vi "Product model selection.vi"(8 "error in (no error)":errorcluster caption="错误输入（无错误）") -> (0 "error in (no error) 2":errorcluster caption="错误输入（无错误）")   [LabVIEW 2017]
uses:
  Picture/SaveButtom.ctl
  Global System.vi
panel:
  out "路径输出":path
  out "添加的路径":path
  in  "Vision Paramter Save Buttom":T1
  out "system time":string
  in  "取消按钮":bool
  in  "确定按钮":bool
  in  "产品处理流程":string(tree)
  in  "产品型号选择":string(combo)
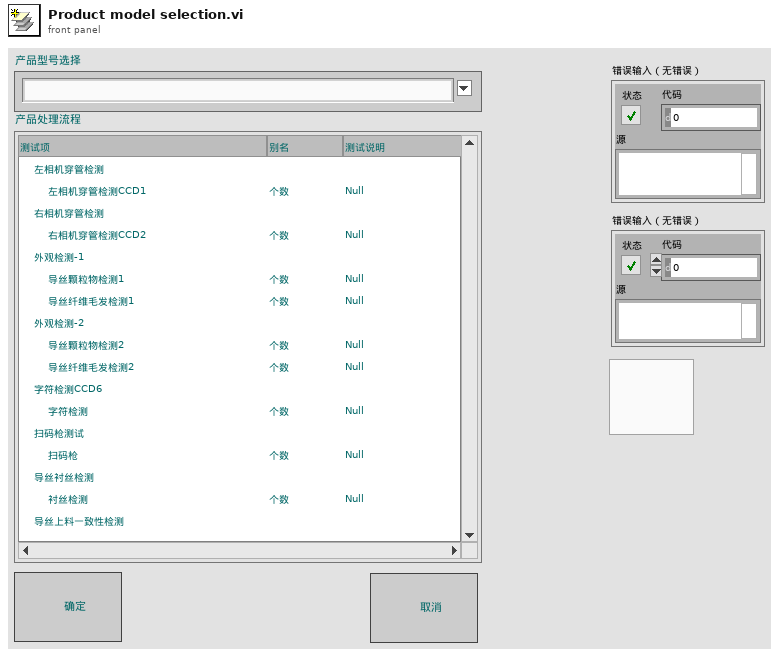
[diagram p1: front panel]
types:
  T1 = typedef "SaveButtom.ctl" = bool
  T2 = cluster{"index":i32, "this vi":refnum<vi>, "error out":errorcluster}
  T3 = cluster{"master data":string, "priority":u16, "secondary data":string[]}
  T4 = cluster{"case name":string[], "queue array":refnum<queue>[]}
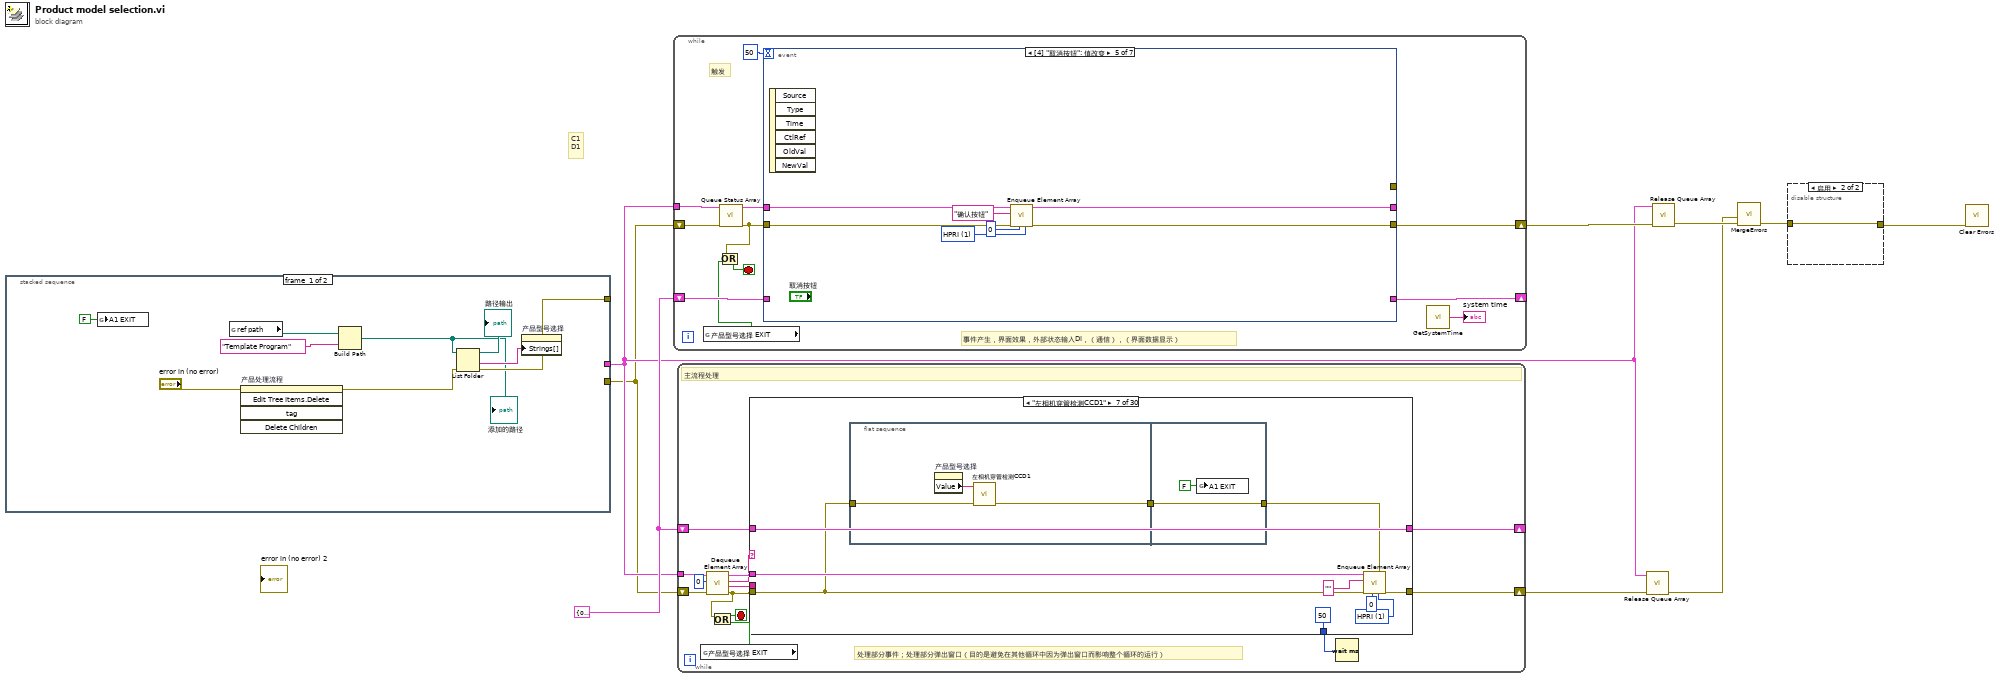
[diagram p0: block diagram]
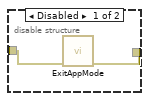
[diagram p2: hidden frame]
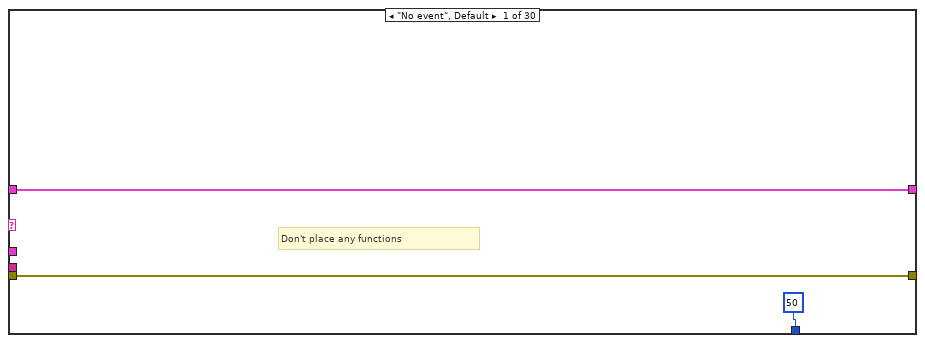
[diagram p3: hidden frame]
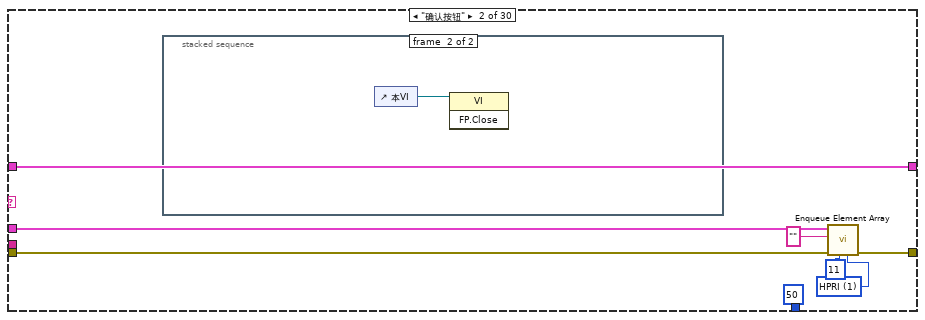
[diagram p4: hidden frame]
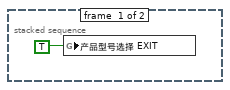
[diagram p5: hidden frame]
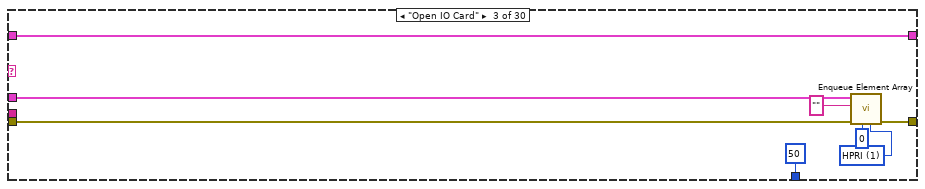
[diagram p6: hidden frame]
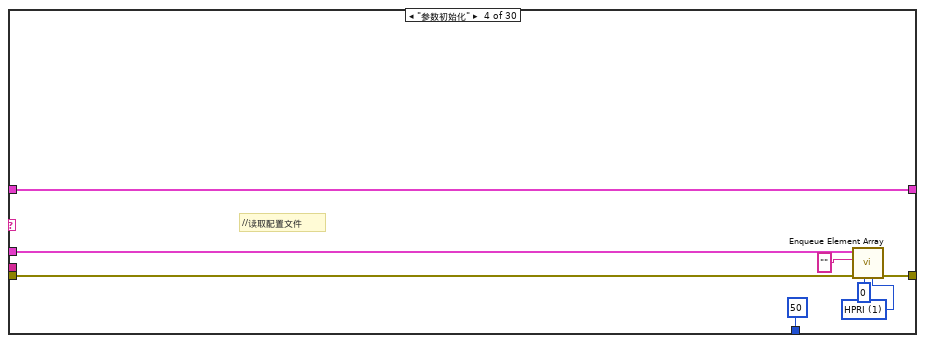
[diagram p7: hidden frame]
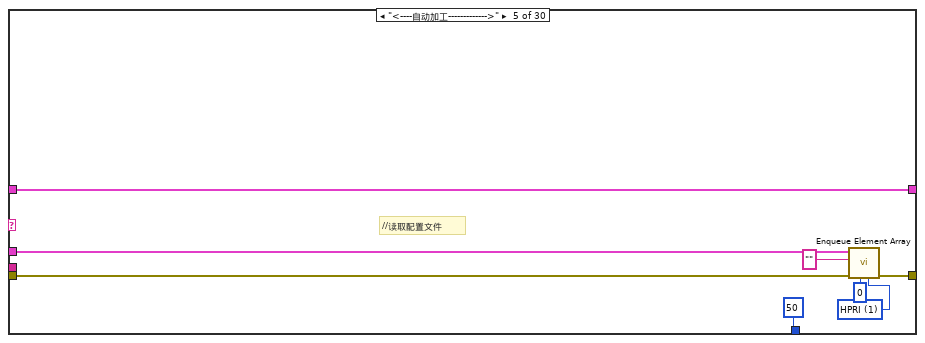
[diagram p8: hidden frame]
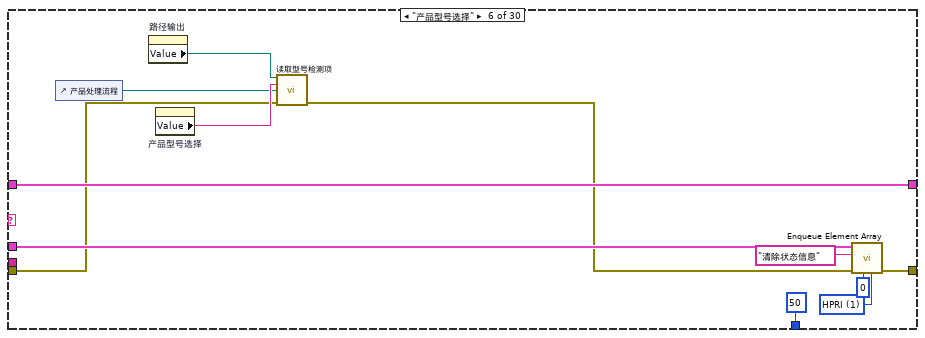
[diagram p9: hidden frame]
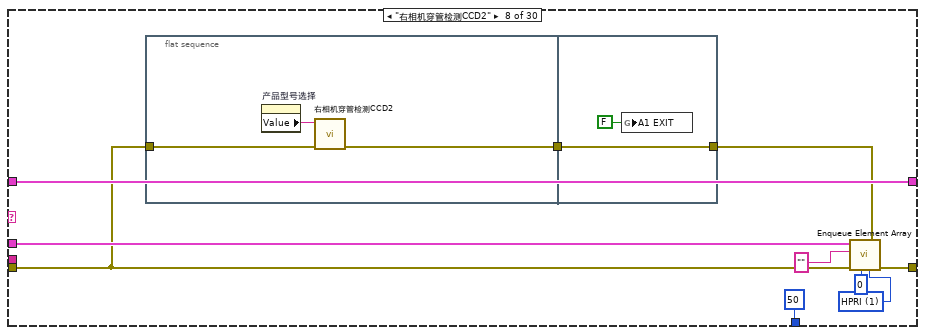
[diagram p10: hidden frame]
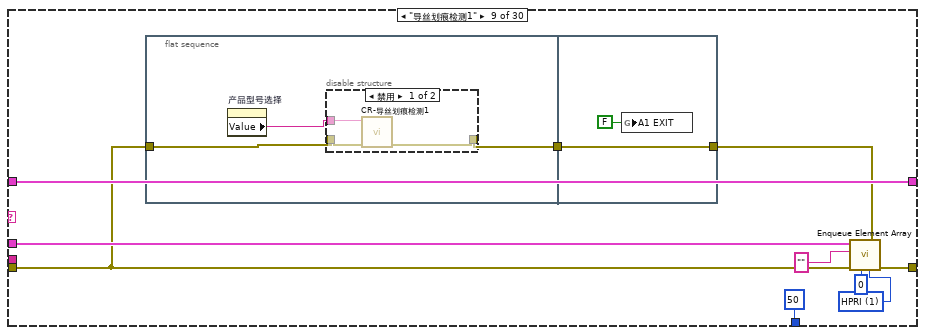
[diagram p11: hidden frame]
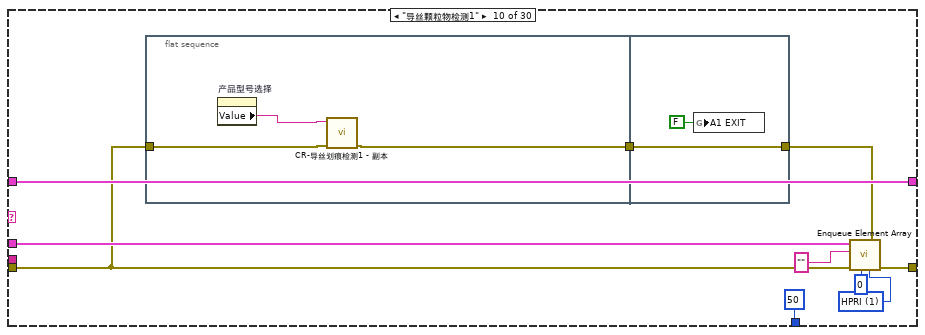
[diagram p13: hidden frame]
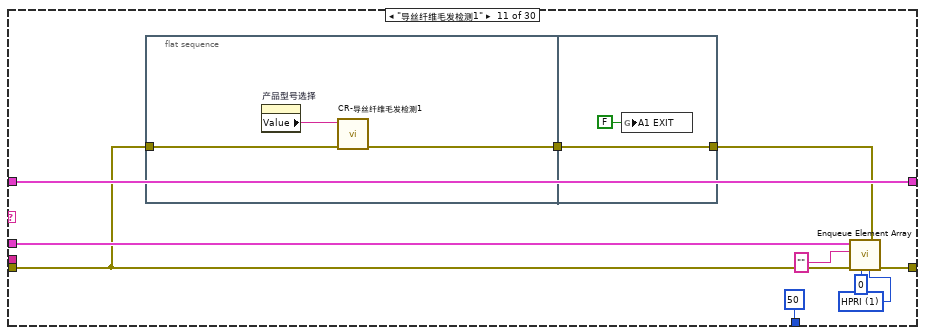
[diagram p14: hidden frame]
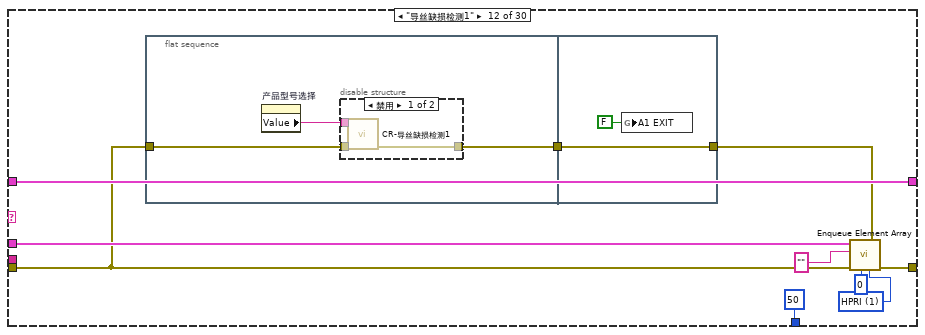
[diagram p15: hidden frame]
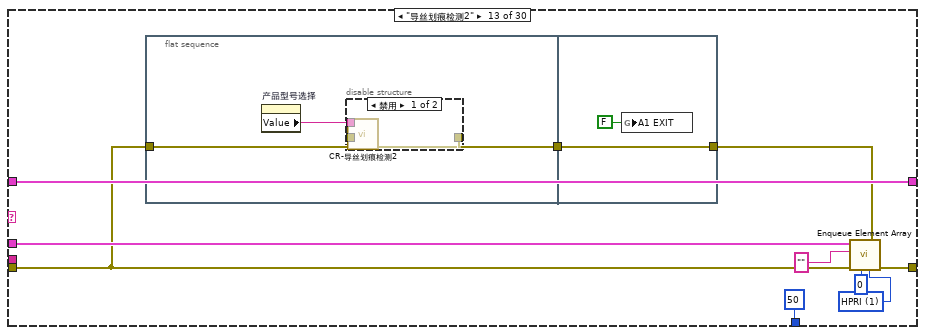
[diagram p17: hidden frame]
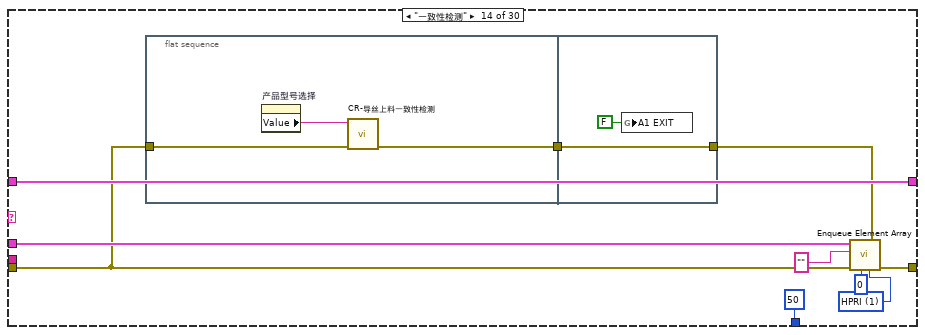
[diagram p19: hidden frame]
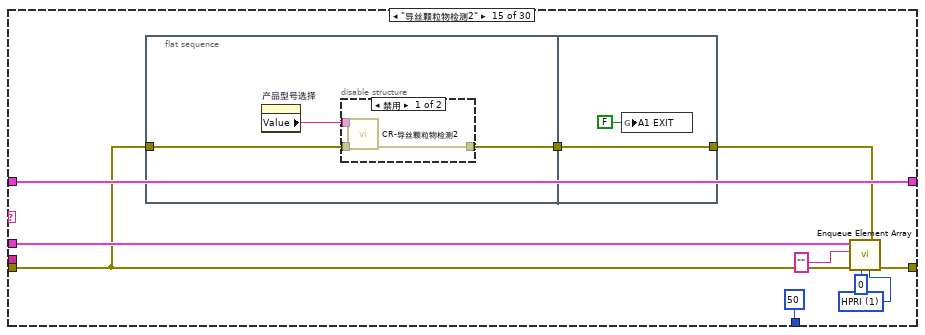
[diagram p20: hidden frame]
diagram:
  w5 = T2 {"index"=0, "this vi"=refnum, "error out"={"status"=FALSE, "code"=0, "source"=""}} ("parameter buffer")
  # "C1\nD1"
  n1 = stacked-sequence {
    tunnel: [w15 _] -> _
    tunnel: [_ w20] -> w1
    tunnel: [_ w19] -> w2
    frame #0 {
      n2 = global write "Global System.vi" "A1 EXIT"(FALSE ("A1 EXIT")) -> ()
      n3 = global read "Global System.vi" "ref path"() -> (w16:path)
      n4 = invoke on="产品处理流程" class="Tree (严格)" method="Edit Tree Items.Delete"(error in="error in (no error)") -> (error out=w11:errorcluster)  [unwired: 4 in, 4 out]
      n5 = Build Path(base path=w16, name or relative path="Template Program" ("名称或相对路径")) -> (appended path=w10:path)
      "添加的路径" <- w10
      n6 = List Folder(path=w10, error in=w11) -> (path out=→"路径输出":path, folder names=w18:string[], error out=w15:errorcluster)  [unwired: 2 in, 1 out]
      n7 = property on="产品型号选择" class="CmbBox"("Strings[]"=w18) -> ()  [unwired: 2 in, 2 out]
    }
    frame #1 {
      w28 = string[] ["comm queue1", "data queue 11", "data queue 12", "data queue 13", "data queue 14"]  # queue name
      w29 = 4  # queue num
      w30 = T3 {"master data"="", "priority"=0, "secondary data"=[]}  # element data type
      n8 = call "Obtain Queue Array.vi"("queue name"=w28, "element data type"=w30, "queue num"=w29) -> ("error out"=w24:errorcluster, "queue out"=w25:T4)  [unwired: 2 in, 1 out]
      n9 = call "Enqueue Element Array.vi"("queue index"=0, "error in"=w24, "master data"="参数初始化", "queue in"=w25) -> ("error out"=w23:errorcluster, "queue out"=w22:T4)  [unwired: 6 in]
      n10 = disable-structure shown="启用" {
        disable-tunnel: w23 -> [w36 w37]
        disable-tunnel: w22 -> [w35 w38]
        disable-tunnel: "Loading Variable" ("master data") -> [w34 _]
        disable-tunnel: [w32 w37] -> w20
        disable-tunnel: [w31 w38] -> w19
        frame Disabled {
          n11 = call "Enqueue Element Array.vi"("queue index"=12, "error in"=w36, "master data"=w34, "queue in"=w35) -> ("error out"=w32:errorcluster, "queue out"=w31:T4)  [unwired: 6 in]
        }
        frame Enabled {
        }
      }
    }
  }
  n12 = while {
    shift-right: [w42] -> w6
    shift-left: w1 -> [w46]
    shift-right: [w44] -> _
    shift-left: w5 -> [w45]
    tunnel: w2 -> [w48]
    stop <- w39 stop-if-true
    # "触发"
    # "事件产生，界面效果，外部状态输入DI，（通信），（界面数据显示）"
    n13 = global read "Global System.vi" "产品型号选择 EXIT"() -> (w40:bool)
    n14 = call "Queue Status Array.vi"("error in (no error)"=w46, "queue in"=w48) -> ("error out"=w41:errorcluster, "queue out"=w43:T4)  [unwired: 4 in]
    n15 = Or(x=w41, y=w40) -> (x .or. y?=w39:bool)
    n16 = event shown="[4] \"取消按钮\": 值改变" {
      selector: _ -> [_ _ _ _ _ _ _]
      dyn-events: _ -> [_ _ _ _ _ _ _]
      timeout: 50 -> [_ _ _ _ _ _ _]
      tunnel: w45 -> [w53 w61 _ _ _ _ _]
      tunnel: [w53 w61 _ _ _ _ _] -> w44
      tunnel: [errorcluster {"status"=FALSE, "code"=0, "source"=""} ("error out") _ _ _ _ _ _] -> _
      tunnel: w43 -> [w51 w60 w66 w73 w80 w87 w95]
      tunnel: w41 -> [w50 w59 w65 w72 w79 w86 w94]
      tunnel: [w50 w58 w63 w70 w77 w84 w92] -> w42
      tunnel: [w51 w57 w64 w71 w78 w85 w93] -> _
      event Timeout {
        # "不要在事件结构里面放入\"弹出窗口\"这样的VI保证该循环畅通无阻。"
        n17 = event-data() -> ()  [unwired: 1 in, 1 out]
      }
      event Panel Close? {
        w55 = u16 1 items=["HPRI"=1, "LPRI"=0] ("priority")
        n18 = event-data() -> ()  [unwired: 1 in, 4 out]
        n19 = call "Enqueue Element Array.vi"("priority"=w55, "queue index"=0, "error in"=w59, "master data"="*Exit application", "queue in"=w60) -> ("error out"=w58:errorcluster, "queue out"=w57:T4)  [unwired: 5 in]
        n20 = event-data("Discard?"=TRUE) -> ()  [unwired: 1 in, 1 out]
      }
      event Value Change {
        w68 = u16 1 items=["HPRI"=1, "LPRI"=0] ("priority")
        n21 = event-data() -> ()  [unwired: 1 in, 6 out]
        n22 = call "Enqueue Element Array.vi"("priority"=w68, "queue index"=0, "error in"=w65, "master data"="Vision Paramter Save", "queue in"=w66) -> ("error out"=w63:errorcluster, "queue out"=w64:T4)  [unwired: 5 in]
      }
      event "确定按钮": Value Change {
        w75 = u16 1 items=["HPRI"=1, "LPRI"=0] ("priority")
        n23 = event-data() -> ()  [unwired: 1 in, 6 out]
        n24 = call "Enqueue Element Array.vi"("priority"=w75, "queue index"=0, "error in"=w72, "master data"="确认按钮", "queue in"=w73) -> ("error out"=w70:errorcluster, "queue out"=w71:T4)  [unwired: 5 in]
      }
      event "取消按钮": Value Change {
        w82 = u16 1 items=["HPRI"=1, "LPRI"=0] ("priority")
        n25 = event-data() -> ()  [unwired: 1 in, 6 out]
        n26 = call "Enqueue Element Array.vi"("priority"=w82, "queue index"=0, "error in"=w79, "master data"="确认按钮", "queue in"=w80) -> ("error out"=w77:errorcluster, "queue out"=w78:T4)  [unwired: 5 in]
      }
      event "产品型号选择": Value Change {
        w89 = u16 1 items=["HPRI"=1, "LPRI"=0] ("priority")
        n27 = event-data() -> ()  [unwired: 1 in, 6 out]
        n28 = call "Enqueue Element Array.vi"("priority"=w89, "queue index"=0, "error in"=w86, "master data"="产品型号选择", "queue in"=w87) -> ("error out"=w84:errorcluster, "queue out"=w85:T4)  [unwired: 5 in]
      }
      event "产品处理流程": Value Change {
        n29 = event-data() -> ("NewVal"=w91:string)  [unwired: 1 in, 5 out]
        n30 = case shown="\"一致性检测\"" w91 {
          tunnel: w95 -> [w97 w104 w111 w118 w125 w132 w139 w146 w153 w160 w167 w174 w181 w188 w195 w202 w209 w216 w223]
          tunnel: w94 -> [w96 w103 w110 w117 w124 w131 w138 w145 w152 w159 w166 w173 w180 w187 w194 w201 w208 w215 w222]
          tunnel: [w97 w102 w109 w116 w123 w130 w137 w144 w151 w158 w165 w172 w179 w186 w193 w200 w207 w214 w221] -> w93
          tunnel: [w96 w101 w108 w115 w122 w129 w136 w143 w150 w157 w164 w171 w178 w185 w192 w199 w206 w213 w220] -> w92
          frame "假", Default {
          }
          frame "左相机穿管检测CCD1" {
            w99 = u16 1 items=["HPRI"=1, "LPRI"=0] ("priority")
            n31 = call "Enqueue Element Array.vi"("priority"=w99, "queue index"=0, "error in"=w103, "master data"="左相机穿管检测CCD1", "queue in"=w104) -> ("error out"=w101:errorcluster, "queue out"=w102:T4)  [unwired: 5 in]
          }
          frame "右相机穿管检测CCD2" {
            w106 = u16 1 items=["HPRI"=1, "LPRI"=0] ("priority")
            n32 = call "Enqueue Element Array.vi"("priority"=w106, "queue index"=0, "error in"=w110, "master data"="右相机穿管检测CCD2", "queue in"=w111) -> ("error out"=w108:errorcluster, "queue out"=w109:T4)  [unwired: 5 in]
          }
          frame "导丝划痕检测1" {
            w113 = u16 1 items=["HPRI"=1, "LPRI"=0] ("priority")
            n33 = call "Enqueue Element Array.vi"("priority"=w113, "queue index"=0, "error in"=w117, "master data"="导丝划痕检测1", "queue in"=w118) -> ("error out"=w115:errorcluster, "queue out"=w116:T4)  [unwired: 5 in]
          }
          frame "导丝颗粒物检测1" {
            w120 = u16 1 items=["HPRI"=1, "LPRI"=0] ("priority")
            n34 = call "Enqueue Element Array.vi"("priority"=w120, "queue index"=0, "error in"=w124, "master data"="导丝颗粒物检测1", "queue in"=w125) -> ("error out"=w122:errorcluster, "queue out"=w123:T4)  [unwired: 5 in]
          }
          frame "导丝纤维毛发检测1" {
            w127 = u16 1 items=["HPRI"=1, "LPRI"=0] ("priority")
            n35 = call "Enqueue Element Array.vi"("priority"=w127, "queue index"=0, "error in"=w131, "master data"="导丝纤维毛发检测1", "queue in"=w132) -> ("error out"=w129:errorcluster, "queue out"=w130:T4)  [unwired: 5 in]
          }
          frame "导丝缺损检测1" {
            w134 = u16 1 items=["HPRI"=1, "LPRI"=0] ("priority")
            n36 = call "Enqueue Element Array.vi"("priority"=w134, "queue index"=0, "error in"=w138, "master data"="导丝缺损检测1", "queue in"=w139) -> ("error out"=w136:errorcluster, "queue out"=w137:T4)  [unwired: 5 in]
          }
          frame "导丝划痕检测2" {
            w141 = u16 1 items=["HPRI"=1, "LPRI"=0] ("priority")
            n37 = call "Enqueue Element Array.vi"("priority"=w141, "queue index"=0, "error in"=w145, "master data"="导丝划痕检测2", "queue in"=w146) -> ("error out"=w143:errorcluster, "queue out"=w144:T4)  [unwired: 5 in]
          }
          frame "导丝颗粒物检测2" {
            w148 = u16 1 items=["HPRI"=1, "LPRI"=0] ("priority")
            n38 = call "Enqueue Element Array.vi"("priority"=w148, "queue index"=0, "error in"=w152, "master data"="导丝颗粒物检测2", "queue in"=w153) -> ("error out"=w150:errorcluster, "queue out"=w151:T4)  [unwired: 5 in]
          }
          frame "导丝纤维毛发检测2" {
            w155 = u16 1 items=["HPRI"=1, "LPRI"=0] ("priority")
            n39 = call "Enqueue Element Array.vi"("priority"=w155, "queue index"=0, "error in"=w159, "master data"="导丝纤维毛发检测2", "queue in"=w160) -> ("error out"=w157:errorcluster, "queue out"=w158:T4)  [unwired: 5 in]
          }
          frame "导丝缺损检测2" {
            w162 = u16 1 items=["HPRI"=1, "LPRI"=0] ("priority")
            n40 = call "Enqueue Element Array.vi"("priority"=w162, "queue index"=0, "error in"=w166, "master data"="导丝缺损检测2", "queue in"=w167) -> ("error out"=w164:errorcluster, "queue out"=w165:T4)  [unwired: 5 in]
          }
          frame "导丝划痕检测3" {
            w169 = u16 1 items=["HPRI"=1, "LPRI"=0] ("priority")
            n41 = call "Enqueue Element Array.vi"("priority"=w169, "queue index"=0, "error in"=w173, "master data"="导丝划痕检测3", "queue in"=w174) -> ("error out"=w171:errorcluster, "queue out"=w172:T4)  [unwired: 5 in]
          }
          frame "导丝颗粒物检测3" {
            w176 = u16 1 items=["HPRI"=1, "LPRI"=0] ("priority")
            n42 = call "Enqueue Element Array.vi"("priority"=w176, "queue index"=0, "error in"=w180, "master data"="导丝颗粒物检测3", "queue in"=w181) -> ("error out"=w178:errorcluster, "queue out"=w179:T4)  [unwired: 5 in]
          }
          frame "导丝纤维毛发检测3" {
            w183 = u16 1 items=["HPRI"=1, "LPRI"=0] ("priority")
            n43 = call "Enqueue Element Array.vi"("priority"=w183, "queue index"=0, "error in"=w187, "master data"="导丝纤维毛发检测3", "queue in"=w188) -> ("error out"=w185:errorcluster, "queue out"=w186:T4)  [unwired: 5 in]
          }
          frame "导丝缺损检测3" {
            w190 = u16 1 items=["HPRI"=1, "LPRI"=0] ("priority")
            n44 = call "Enqueue Element Array.vi"("priority"=w190, "queue index"=0, "error in"=w194, "master data"="导丝缺损检测3", "queue in"=w195) -> ("error out"=w192:errorcluster, "queue out"=w193:T4)  [unwired: 5 in]
          }
          frame "字符检测" {
            w197 = u16 1 items=["HPRI"=1, "LPRI"=0] ("priority")
            n45 = call "Enqueue Element Array.vi"("priority"=w197, "queue index"=0, "error in"=w201, "master data"="字符检测", "queue in"=w202) -> ("error out"=w199:errorcluster, "queue out"=w200:T4)  [unwired: 5 in]
          }
          frame "扫码枪" {
            w204 = u16 1 items=["HPRI"=1, "LPRI"=0] ("priority")
            n46 = call "Enqueue Element Array.vi"("priority"=w204, "queue index"=0, "error in"=w208, "master data"="扫码枪扫码", "queue in"=w209) -> ("error out"=w206:errorcluster, "queue out"=w207:T4)  [unwired: 5 in]
          }
          frame "衬丝检测" {
            w211 = u16 1 items=["HPRI"=1, "LPRI"=0] ("priority")
            n47 = call "Enqueue Element Array.vi"("priority"=w211, "queue index"=0, "error in"=w215, "master data"="衬丝检测", "queue in"=w216) -> ("error out"=w213:errorcluster, "queue out"=w214:T4)  [unwired: 5 in]
          }
          frame "一致性检测" {
            w218 = u16 1 items=["HPRI"=1, "LPRI"=0] ("priority")
            n48 = call "Enqueue Element Array.vi"("priority"=w218, "queue index"=0, "error in"=w222, "master data"="一致性检测", "queue in"=w223) -> ("error out"=w220:errorcluster, "queue out"=w221:T4)  [unwired: 5 in]
          }
        }
      }
    }
    n49 = call "GetSystemTime.vi"() -> ("date/time string"=→"system time":string)  [unwired: 7 in]
  }
  n50 = while {
    shift-right: [w236] -> w4
    shift-left: w1 -> [w227]
    shift-right: [w233] -> _
    shift-left: w5 -> [w234]
    tunnel: w2 -> [w229]
    stop <- w224 stop-if-true
    # "处理部分事件；处理部分弹出窗口（目的是避免在其他循环中因为弹出窗口而影响整个循环的运行）"
    # "主流程处理"
    n51 = global read "Global System.vi" "产品型号选择 EXIT"() -> (w225:bool)
    n52 = call "Dequeue Element Array.vi"("queue in"=w229, "queue index"=0, "error in"=w227) -> ("queue out"=w232:T4, "master data"=w231:string, "secondary data"=w230:string[], "error out"=w226:errorcluster)  [unwired: 2 in, 1 out]
    n53 = Or(x=w226, y=w225) -> (x .or. y?=w224:bool)
    n54 = case shown="\"左相机穿管检测CCD1\"" w231 {
      tunnel: w232 -> [_ w246 w256 w264 w272 w279 w294 w309 w324 w342 w357 w372 w390 w408 w423 w441 w459 w477 w495 w513 w531 w549 w564 w579 w592 w600 w608 w616 w624 w630]
      tunnel: w226 -> [w238 w242 w252 w261 w268 w275 w288 w303 w318 w336 w351 w366 w384 w402 w417 w435 w453 w471 w489 w507 w525 w543 w558 w573 w587 w596 w604 w612 w620 w627]
      tunnel: [w238 w245 w255 w263 w271 w284 w293 w308 w323 w341 w356 w371 w389 w407 w422 w440 w458 w476 w494 w512 w530 w548 w563 w578 w591 w599 w607 w615 w623 w638] -> w236
      tunnel: [50 50 50 50 50 50 50 50 50 50 50 50 50 50 50 50 50 50 50 50 50 50 50 50 50 50 50 50 50 50] -> w235
      tunnel: w234 -> [w239 w243 w253 w258 w269 w280 w289 w304 w319 w337 w352 w367 w385 w403 w418 w436 w454 w472 w490 w508 w526 w544 w559 w574 w586 w597 w605 w613 w621 w636]
      tunnel: [w239 w243 w253 w258 w269 w280 w289 w304 w319 w337 w352 w367 w385 w403 w418 w436 w454 w472 w490 w508 w526 w544 w559 w574 w586 w597 w605 w613 w621 w636] -> w233
      tunnel: w230 -> [_ _ _ _ _ _ _ _ _ _ _ _ _ _ _ _ _ _ _ _ _ _ _ _ _ _ _ _ _ _]
      frame "No event", Default {
        # "Don't place any functions"
      }
      frame "确认按钮" {
        w240 = u16 1 items=["HPRI"=1, "LPRI"=0] ("priority")
        n55 = stacked-sequence {
          frame #0 {
            n56 = global write "Global System.vi" "产品型号选择 EXIT"(TRUE ("EXIT")) -> ()
          }
          frame #1 {
            n57 = control-ref of="本VI"() -> (w249:refnum<vi>)
            n58 = invoke class="VI" method="FP.Close"(reference=w249) -> ()  [unwired: 2 in, 3 out]
          }
        }
        n59 = call "Enqueue Element Array.vi"("priority"=w240, "queue index"=11, "error in"=w242, "master data"="" ("Element 1"), "queue in"=w246) -> ("error out"=w245:errorcluster)  [unwired: 5 in, 1 out]
      }
      frame "Open IO Card" {
        w250 = u16 1 items=["HPRI"=1, "LPRI"=0] ("priority")
        n60 = call "Enqueue Element Array.vi"("priority"=w250, "queue index"=0, "error in"=w252, "master data"="" ("Element 1"), "queue in"=w256) -> ("error out"=w255:errorcluster)  [unwired: 5 in, 1 out]
      }
      frame "参数初始化" {
        w259 = u16 1 items=["HPRI"=1, "LPRI"=0] ("priority")
        # "//读取配置文件"
        n61 = call "Enqueue Element Array.vi"("priority"=w259, "queue index"=0, "error in"=w261, "master data"="" ("Element 1"), "queue in"=w264) -> ("error out"=w263:errorcluster)  [unwired: 5 in, 1 out]
      }
      frame "<----自动加工------------->" {
        w266 = u16 1 items=["HPRI"=1, "LPRI"=0] ("priority")
        # "//读取配置文件"
        n62 = call "Enqueue Element Array.vi"("priority"=w266, "queue index"=0, "error in"=w268, "master data"="" ("Element 1"), "queue in"=w272) -> ("error out"=w271:errorcluster)  [unwired: 5 in, 1 out]
      }
      frame "产品型号选择" {
        w281 = u16 1 items=["HPRI"=1, "LPRI"=0] ("priority")
        n63 = control-ref of="产品处理流程"() -> (w276:refnum<vi>)
        n64 = property on="路径输出" class="Path"() -> ("Value"=w278:path)  [unwired: 2 in, 2 out]
        n65 = property on="产品型号选择" class="CmbBox"() -> ("Value"=w277:string)  [unwired: 2 in, 2 out]
        n66 = call "读取型号检测项.vi"("产品型号路径"=w278, "产品型号"=w277, "树形List"=w276, "error in (no error)"=w275) -> ("error out"=w274:errorcluster)  [unwired: 11 in]
        n67 = call "Enqueue Element Array.vi"("priority"=w281, "queue index"=0, "error in"=w274, "master data"="清除状态信息" ("Element 1"), "queue in"=w279) -> ("error out"=w284:errorcluster)  [unwired: 5 in, 1 out]
      }
      frame "左相机穿管检测CCD1" {
        w290 = u16 1 items=["HPRI"=1, "LPRI"=0] ("priority")
        n68 = flat-sequence {
          tunnel: w288 -> [w298]
          tunnel: [w297] -> w286
          tunnel: [w299] -> w287
          tunnel: w286 -> [w299]
          frame #0 {
            n69 = property on="产品型号选择" class="CmbBox"() -> ("Value"=w296:string)  [unwired: 2 in, 2 out]
            n70 = call "左相机穿管检测CCD1.vi"("error in (no error)"=w298, "名称或相对路径"=w296) -> ("error in (no error) 2"=w297:errorcluster)  [unwired: 9 in]
          }
          frame #1 {
            n71 = global write "Global System.vi" "A1 EXIT"(FALSE ("A1 EXIT")) -> ()
          }
        }
        n72 = call "Enqueue Element Array.vi"("priority"=w290, "device error in"=w287, "queue index"=0, "error in"=w288, "master data"="" ("Element 1"), "queue in"=w294) -> ("error out"=w293:errorcluster)  [unwired: 4 in, 1 out]
      }
      frame "右相机穿管检测CCD2" {
        w305 = u16 1 items=["HPRI"=1, "LPRI"=0] ("priority")
        n73 = flat-sequence {
          tunnel: w303 -> [w313]
          tunnel: [w312] -> w301
          tunnel: [w314] -> w302
          tunnel: w301 -> [w314]
          frame #0 {
            n74 = property on="产品型号选择" class="CmbBox"() -> ("Value"=w311:string)  [unwired: 2 in, 2 out]
            n75 = call "右相机穿管检测CCD2.vi"("error in (no error)"=w313, "名称或相对路径"=w311) -> ("error in (no error) 2"=w312:errorcluster)  [unwired: 9 in]
          }
          frame #1 {
            n76 = global write "Global System.vi" "A1 EXIT"(FALSE ("A1 EXIT")) -> ()
          }
        }
        n77 = call "Enqueue Element Array.vi"("priority"=w305, "device error in"=w302, "queue index"=0, "error in"=w303, "master data"="" ("Element 1"), "queue in"=w309) -> ("error out"=w308:errorcluster)  [unwired: 4 in, 1 out]
      }
      frame "导丝划痕检测1" {
        w320 = u16 1 items=["HPRI"=1, "LPRI"=0] ("priority")
        n78 = flat-sequence {
          tunnel: w318 -> [w328]
          tunnel: [w327] -> w316
          tunnel: [w332] -> w317
          tunnel: w316 -> [w332]
          frame #0 {
            n79 = property on="产品型号选择" class="CmbBox"() -> ("Value"=w326:string)  [unwired: 2 in, 2 out]
            n80 = disable-structure shown="禁用" {
              disable-tunnel: w328 -> [w331 _]
              disable-tunnel: [w330 _] -> w327
              disable-tunnel: w326 -> [w329 _]
              frame Disabled {
                n81 = call "CR-导丝划痕检测1.vi"("error in (no error)"=w331, "名称或相对路径"=w329) -> ("error in (no error) 2"=w330:errorcluster)  [unwired: 9 in]
              }
              frame Enabled {
              }
            }
          }
          frame #1 {
            n82 = global write "Global System.vi" "A1 EXIT"(FALSE ("A1 EXIT")) -> ()
          }
        }
        n83 = call "Enqueue Element Array.vi"("priority"=w320, "device error in"=w317, "queue index"=0, "error in"=w318, "master data"="" ("Element 1"), "queue in"=w324) -> ("error out"=w323:errorcluster)  [unwired: 4 in, 1 out]
      }
      frame "导丝颗粒物检测1" {
        w338 = u16 1 items=["HPRI"=1, "LPRI"=0] ("priority")
        n84 = flat-sequence {
          tunnel: w336 -> [w346]
          tunnel: [w345] -> w334
          tunnel: [w347] -> w335
          tunnel: w334 -> [w347]
          frame #0 {
            n85 = property on="产品型号选择" class="CmbBox"() -> ("Value"=w344:string)  [unwired: 2 in, 2 out]
            n86 = call "CR-导丝划痕检测1 - 副本.vi"("error in (no error)"=w346, "名称或相对路径"=w344) -> ("error in (no error) 2"=w345:errorcluster)  [unwired: 9 in]
          }
          frame #1 {
            n87 = global write "Global System.vi" "A1 EXIT"(FALSE ("A1 EXIT")) -> ()
          }
        }
        n88 = call "Enqueue Element Array.vi"("priority"=w338, "device error in"=w335, "queue index"=0, "error in"=w336, "master data"="" ("Element 1"), "queue in"=w342) -> ("error out"=w341:errorcluster)  [unwired: 4 in, 1 out]
      }
      frame "导丝纤维毛发检测1" {
        w353 = u16 1 items=["HPRI"=1, "LPRI"=0] ("priority")
        n89 = flat-sequence {
          tunnel: w351 -> [w361]
          tunnel: [w360] -> w349
          tunnel: [w362] -> w350
          tunnel: w349 -> [w362]
          frame #0 {
            n90 = property on="产品型号选择" class="CmbBox"() -> ("Value"=w359:string)  [unwired: 2 in, 2 out]
            n91 = call "CR-导丝纤维毛发检测1.vi"("error in (no error)"=w361, "名称或相对路径"=w359) -> ("error in (no error) 2"=w360:errorcluster)  [unwired: 9 in]
          }
          frame #1 {
            n92 = global write "Global System.vi" "A1 EXIT"(FALSE ("A1 EXIT")) -> ()
          }
        }
        n93 = call "Enqueue Element Array.vi"("priority"=w353, "device error in"=w350, "queue index"=0, "error in"=w351, "master data"="" ("Element 1"), "queue in"=w357) -> ("error out"=w356:errorcluster)  [unwired: 4 in, 1 out]
      }
      frame "导丝缺损检测1" {
        w368 = u16 1 items=["HPRI"=1, "LPRI"=0] ("priority")
        n94 = flat-sequence {
          tunnel: w366 -> [w376]
          tunnel: [w375] -> w364
          tunnel: [w380] -> w365
          tunnel: w364 -> [w380]
          frame #0 {
            n95 = property on="产品型号选择" class="CmbBox"() -> ("Value"=w374:string)  [unwired: 2 in, 2 out]
            n96 = disable-structure shown="禁用" {
              disable-tunnel: w376 -> [w379 _]
              disable-tunnel: [w378 _] -> w375
              disable-tunnel: w374 -> [w377 _]
              frame Disabled {
                n97 = call "CR-导丝缺损检测1.vi"("error in (no error)"=w379, "名称或相对路径"=w377) -> ("error in (no error) 2"=w378:errorcluster)  [unwired: 9 in]
              }
              frame Enabled {
              }
            }
          }
          frame #1 {
            n98 = global write "Global System.vi" "A1 EXIT"(FALSE ("A1 EXIT")) -> ()
          }
        }
        n99 = call "Enqueue Element Array.vi"("priority"=w368, "device error in"=w365, "queue index"=0, "error in"=w366, "master data"="" ("Element 1"), "queue in"=w372) -> ("error out"=w371:errorcluster)  [unwired: 4 in, 1 out]
      }
      frame "导丝划痕检测2" {
        w386 = u16 1 items=["HPRI"=1, "LPRI"=0] ("priority")
        n100 = flat-sequence {
          tunnel: w384 -> [w394]
          tunnel: [w393] -> w382
          tunnel: [w398] -> w383
          tunnel: w382 -> [w398]
          frame #0 {
            n101 = property on="产品型号选择" class="CmbBox"() -> ("Value"=w392:string)  [unwired: 2 in, 2 out]
            n102 = disable-structure shown="禁用" {
              disable-tunnel: w394 -> [w397 _]
              disable-tunnel: [w396 _] -> w393
              disable-tunnel: w392 -> [w395 _]
              frame Disabled {
                n103 = call "CR-导丝划痕检测2.vi"("error in (no error)"=w397, "名称或相对路径"=w395) -> ("error in (no error) 2"=w396:errorcluster)  [unwired: 9 in]
              }
              frame Enabled {
              }
            }
          }
          frame #1 {
            n104 = global write "Global System.vi" "A1 EXIT"(FALSE ("A1 EXIT")) -> ()
          }
        }
        n105 = call "Enqueue Element Array.vi"("priority"=w386, "device error in"=w383, "queue index"=0, "error in"=w384, "master data"="" ("Element 1"), "queue in"=w390) -> ("error out"=w389:errorcluster)  [unwired: 4 in, 1 out]
      }
      frame "一致性检测" {
        w404 = u16 1 items=["HPRI"=1, "LPRI"=0] ("priority")
        n106 = flat-sequence {
          tunnel: w402 -> [w412]
          tunnel: [w411] -> w400
          tunnel: [w413] -> w401
          tunnel: w400 -> [w413]
          frame #0 {
            n107 = property on="产品型号选择" class="CmbBox"() -> ("Value"=w410:string)  [unwired: 2 in, 2 out]
            n108 = call "CR-导丝上料一致性检测.vi"("error in (no error)"=w412, "名称或相对路径"=w410) -> ("error in (no error) 2"=w411:errorcluster)  [unwired: 9 in]
          }
          frame #1 {
            n109 = global write "Global System.vi" "A1 EXIT"(FALSE ("A1 EXIT")) -> ()
          }
        }
        n110 = call "Enqueue Element Array.vi"("priority"=w404, "device error in"=w401, "queue index"=0, "error in"=w402, "master data"="" ("Element 1"), "queue in"=w408) -> ("error out"=w407:errorcluster)  [unwired: 4 in, 1 out]
      }
      frame "导丝颗粒物检测2" {
        w419 = u16 1 items=["HPRI"=1, "LPRI"=0] ("priority")
        n111 = flat-sequence {
          tunnel: w417 -> [w427]
          tunnel: [w426] -> w415
          tunnel: [w431] -> w416
          tunnel: w415 -> [w431]
          frame #0 {
            n112 = property on="产品型号选择" class="CmbBox"() -> ("Value"=w425:string)  [unwired: 2 in, 2 out]
            n113 = disable-structure shown="禁用" {
              disable-tunnel: w427 -> [w430 _]
              disable-tunnel: [w429 _] -> w426
              disable-tunnel: w425 -> [w428 _]
              frame Disabled {
                n114 = call "CR-导丝颗粒物检测2.vi"("error in (no error)"=w430, "名称或相对路径"=w428) -> ("error in (no error) 2"=w429:errorcluster)  [unwired: 9 in]
              }
              frame Enabled {
              }
            }
          }
          frame #1 {
            n115 = global write "Global System.vi" "A1 EXIT"(FALSE ("A1 EXIT")) -> ()
          }
        }
        n116 = call "Enqueue Element Array.vi"("priority"=w419, "device error in"=w416, "queue index"=0, "error in"=w417, "master data"="" ("Element 1"), "queue in"=w423) -> ("error out"=w422:errorcluster)  [unwired: 4 in, 1 out]
      }
      frame "导丝纤维毛发检测2" {
        w437 = u16 1 items=["HPRI"=1, "LPRI"=0] ("priority")
        n117 = flat-sequence {
          tunnel: w435 -> [w445]
          tunnel: [w444] -> w433
          tunnel: [w449] -> w434
          tunnel: w433 -> [w449]
          frame #0 {
            n118 = property on="产品型号选择" class="CmbBox"() -> ("Value"=w443:string)  [unwired: 2 in, 2 out]
            n119 = disable-structure shown="禁用" {
              disable-tunnel: w445 -> [w448 _]
              disable-tunnel: [w447 _] -> w444
              disable-tunnel: w443 -> [w446 _]
              frame Disabled {
                n120 = call "CR-导丝纤维毛发检测2.vi"("error in (no error)"=w448, "名称或相对路径"=w446) -> ("error in (no error) 2"=w447:errorcluster)  [unwired: 9 in]
              }
              frame Enabled {
              }
            }
          }
          frame #1 {
            n121 = global write "Global System.vi" "A1 EXIT"(FALSE ("A1 EXIT")) -> ()
          }
        }
        n122 = call "Enqueue Element Array.vi"("priority"=w437, "device error in"=w434, "queue index"=0, "error in"=w435, "master data"="" ("Element 1"), "queue in"=w441) -> ("error out"=w440:errorcluster)  [unwired: 4 in, 1 out]
      }
      frame "导丝缺损检测2" {
        w455 = u16 1 items=["HPRI"=1, "LPRI"=0] ("priority")
        n123 = flat-sequence {
          tunnel: w453 -> [w463]
          tunnel: [w462] -> w451
          tunnel: [w467] -> w452
          tunnel: w451 -> [w467]
          frame #0 {
            n124 = property on="产品型号选择" class="CmbBox"() -> ("Value"=w461:string)  [unwired: 2 in, 2 out]
            n125 = disable-structure shown="禁用" {
              disable-tunnel: w463 -> [w466 _]
              disable-tunnel: [w465 _] -> w462
              disable-tunnel: w461 -> [w464 _]
              frame Disabled {
                n126 = call "CR-导丝缺损检测2.vi"("error in (no error)"=w466, "名称或相对路径"=w464) -> ("error in (no error) 2"=w465:errorcluster)  [unwired: 9 in]
              }
              frame Enabled {
              }
            }
          }
          frame #1 {
            n127 = global write "Global System.vi" "A1 EXIT"(FALSE ("A1 EXIT")) -> ()
          }
        }
        n128 = call "Enqueue Element Array.vi"("priority"=w455, "device error in"=w452, "queue index"=0, "error in"=w453, "master data"="" ("Element 1"), "queue in"=w459) -> ("error out"=w458:errorcluster)  [unwired: 4 in, 1 out]
      }
      frame "导丝划痕检测3" {
        w473 = u16 1 items=["HPRI"=1, "LPRI"=0] ("priority")
        n129 = flat-sequence {
          tunnel: w471 -> [w481]
          tunnel: [w480] -> w469
          tunnel: [w485] -> w470
          tunnel: w469 -> [w485]
          frame #0 {
            n130 = property on="产品型号选择" class="CmbBox"() -> ("Value"=w479:string)  [unwired: 2 in, 2 out]
            n131 = disable-structure shown="禁用" {
              disable-tunnel: w481 -> [w484 _]
              disable-tunnel: [w483 _] -> w480
              disable-tunnel: w479 -> [w482 _]
              frame Disabled {
                n132 = call "CR-导丝划痕检测3.vi"("error in (no error)"=w484, "名称或相对路径"=w482) -> ("error in (no error) 2"=w483:errorcluster)  [unwired: 9 in]
              }
              frame Enabled {
              }
            }
          }
          frame #1 {
            n133 = global write "Global System.vi" "A1 EXIT"(FALSE ("A1 EXIT")) -> ()
          }
        }
        n134 = call "Enqueue Element Array.vi"("priority"=w473, "device error in"=w470, "queue index"=0, "error in"=w471, "master data"="" ("Element 1"), "queue in"=w477) -> ("error out"=w476:errorcluster)  [unwired: 4 in, 1 out]
      }
      frame "导丝颗粒物检测3" {
        w491 = u16 1 items=["HPRI"=1, "LPRI"=0] ("priority")
        n135 = flat-sequence {
          tunnel: w489 -> [w499]
          tunnel: [w498] -> w487
          tunnel: [w503] -> w488
          tunnel: w487 -> [w503]
          frame #0 {
            n136 = property on="产品型号选择" class="CmbBox"() -> ("Value"=w497:string)  [unwired: 2 in, 2 out]
            n137 = disable-structure shown="禁用" {
              disable-tunnel: w499 -> [w502 _]
              disable-tunnel: [w501 _] -> w498
              disable-tunnel: w497 -> [w500 _]
              frame Disabled {
                n138 = call "CR-导丝颗粒物检测3.vi"("error in (no error)"=w502, "名称或相对路径"=w500) -> ("error in (no error) 2"=w501:errorcluster)  [unwired: 9 in]
              }
              frame Enabled {
              }
            }
          }
          frame #1 {
            n139 = global write "Global System.vi" "A1 EXIT"(FALSE ("A1 EXIT")) -> ()
          }
        }
        n140 = call "Enqueue Element Array.vi"("priority"=w491, "device error in"=w488, "queue index"=0, "error in"=w489, "master data"="" ("Element 1"), "queue in"=w495) -> ("error out"=w494:errorcluster)  [unwired: 4 in, 1 out]
      }
      frame "导丝纤维毛发检测3" {
        w509 = u16 1 items=["HPRI"=1, "LPRI"=0] ("priority")
        n141 = flat-sequence {
          tunnel: w507 -> [w517]
          tunnel: [w516] -> w505
          tunnel: [w521] -> w506
          tunnel: w505 -> [w521]
          frame #0 {
            n142 = property on="产品型号选择" class="CmbBox"() -> ("Value"=w515:string)  [unwired: 2 in, 2 out]
            n143 = disable-structure shown="禁用" {
              disable-tunnel: w517 -> [w520 _]
              disable-tunnel: [w519 _] -> w516
              disable-tunnel: w515 -> [w518 _]
              frame Disabled {
                n144 = call "CR-导丝纤维毛发检测3.vi"("error in (no error)"=w520, "名称或相对路径"=w518) -> ("error in (no error) 2"=w519:errorcluster)  [unwired: 9 in]
              }
              frame Enabled {
              }
            }
          }
          frame #1 {
            n145 = global write "Global System.vi" "A1 EXIT"(FALSE ("A1 EXIT")) -> ()
          }
        }
        n146 = call "Enqueue Element Array.vi"("priority"=w509, "device error in"=w506, "queue index"=0, "error in"=w507, "master data"="" ("Element 1"), "queue in"=w513) -> ("error out"=w512:errorcluster)  [unwired: 4 in, 1 out]
      }
      frame "导丝缺损检测3" {
        w527 = u16 1 items=["HPRI"=1, "LPRI"=0] ("priority")
        n147 = flat-sequence {
          tunnel: w525 -> [w535]
          tunnel: [w534] -> w523
          tunnel: [w539] -> w524
          tunnel: w523 -> [w539]
          frame #0 {
            n148 = property on="产品型号选择" class="CmbBox"() -> ("Value"=w533:string)  [unwired: 2 in, 2 out]
            n149 = disable-structure shown="禁用" {
              disable-tunnel: w535 -> [w538 _]
              disable-tunnel: [w537 _] -> w534
              disable-tunnel: w533 -> [w536 _]
              frame Disabled {
                n150 = call "CR-导丝缺损检测3.vi"("error in (no error)"=w538, "名称或相对路径"=w536) -> ("error in (no error) 2"=w537:errorcluster)  [unwired: 9 in]
              }
              frame Enabled {
              }
            }
          }
          frame #1 {
            n151 = global write "Global System.vi" "A1 EXIT"(FALSE ("A1 EXIT")) -> ()
          }
        }
        n152 = call "Enqueue Element Array.vi"("priority"=w527, "device error in"=w524, "queue index"=0, "error in"=w525, "master data"="" ("Element 1"), "queue in"=w531) -> ("error out"=w530:errorcluster)  [unwired: 4 in, 1 out]
      }
      frame "字符检测" {
        w545 = u16 1 items=["HPRI"=1, "LPRI"=0] ("priority")
        n153 = flat-sequence {
          tunnel: w543 -> [w553]
          tunnel: [w552] -> w541
          tunnel: [w554] -> w542
          tunnel: w541 -> [w554]
          frame #0 {
            n154 = property on="产品型号选择" class="CmbBox"() -> ("Value"=w551:string)  [unwired: 2 in, 2 out]
            n155 = call "CR-字符串检测CCD6.vi"("error in (no error)"=w553, "名称或相对路径"=w551) -> ("error in (no error) 2"=w552:errorcluster)  [unwired: 9 in]
          }
          frame #1 {
            n156 = global write "Global System.vi" "A1 EXIT"(FALSE ("A1 EXIT")) -> ()
          }
        }
        n157 = call "Enqueue Element Array.vi"("priority"=w545, "device error in"=w542, "queue index"=0, "error in"=w543, "master data"="" ("Element 1"), "queue in"=w549) -> ("error out"=w548:errorcluster)  [unwired: 4 in, 1 out]
      }
      frame "衬丝检测" {
        w560 = u16 1 items=["HPRI"=1, "LPRI"=0] ("priority")
        n158 = flat-sequence {
          tunnel: w558 -> [w568]
          tunnel: [w567] -> w556
          tunnel: [w569] -> w557
          tunnel: w556 -> [w569]
          frame #0 {
            n159 = property on="产品型号选择" class="CmbBox"() -> ("Value"=w566:string)  [unwired: 2 in, 2 out]
            n160 = call "CR-字符串检测衬丝.vi"("error in (no error)"=w568, "名称或相对路径"=w566) -> ("error in (no error) 2"=w567:errorcluster)  [unwired: 9 in]
          }
          frame #1 {
            n161 = global write "Global System.vi" "A1 EXIT"(FALSE ("A1 EXIT")) -> ()
          }
        }
        n162 = call "Enqueue Element Array.vi"("priority"=w560, "device error in"=w557, "queue index"=0, "error in"=w558, "master data"="" ("Element 1"), "queue in"=w564) -> ("error out"=w563:errorcluster)  [unwired: 4 in, 1 out]
      }
      frame "扫码枪扫码" {
        w575 = u16 1 items=["HPRI"=1, "LPRI"=0] ("priority")
        n163 = flat-sequence {
          tunnel: w573 -> [w582]
          tunnel: [w581] -> w571
          tunnel: [w584] -> w572
          tunnel: w571 -> [w584]
          frame #0 {
            n164 = property on="产品型号选择" class="CmbBox"() -> ("Value"=w583:string)  [unwired: 2 in, 2 out]
            n165 = call "CR-扫码枪.vi"("error in (no error)"=w582, "名称或相对路径"=w583) -> ("error in (no error) 2"=w581:errorcluster)  [unwired: 9 in]
          }
          frame #1 {
            n166 = global write "Global System.vi" "A1 EXIT"(FALSE ("A1 EXIT")) -> ()
          }
        }
        n167 = call "Enqueue Element Array.vi"("priority"=w575, "device error in"=w572, "queue index"=0, "error in"=w573, "master data"="" ("Element 1"), "queue in"=w579) -> ("error out"=w578:errorcluster)  [unwired: 4 in, 1 out]
      }
      frame "IOandPos Updata" {
        w589 = u16 0 items=["HPRI"=1, "LPRI"=0] ("priority")
        n168 = call "Enqueue Element Array.vi"("priority"=w589, "queue index"=1, "error in"=w587, "master data"="IOandPos Updata", "queue in"=w592) -> ("error out"=w591:errorcluster)  [unwired: 5 in, 1 out]
      }
      frame "<-----自动加工结束--------->" {
        w594 = u16 1 items=["HPRI"=1, "LPRI"=0] ("priority")
        # "//读取配置文件"
        n169 = call "Enqueue Element Array.vi"("priority"=w594, "queue index"=1, "error in"=w596, "master data"="" ("Element 1"), "queue in"=w600) -> ("error out"=w599:errorcluster)  [unwired: 5 in, 1 out]
      }
      frame "<----------手动部分------------->" {
        w602 = u16 1 items=["HPRI"=1, "LPRI"=0] ("priority")
        # "//读取配置文件"
        n170 = call "Enqueue Element Array.vi"("priority"=w602, "queue index"=1, "error in"=w604, "master data"="" ("Element 1"), "queue in"=w608) -> ("error out"=w607:errorcluster)  [unwired: 5 in, 1 out]
      }
      frame "参数设置保存" {
        w610 = u16 1 items=["HPRI"=1, "LPRI"=0] ("priority")
        n171 = call "Enqueue Element Array.vi"("priority"=w610, "queue index"=1, "error in"=w612, "master data"="" ("Element 1"), "queue in"=w616) -> ("error out"=w615:errorcluster)  [unwired: 5 in, 1 out]
      }
      frame "<--------------手动结束---------------->" {
        w618 = u16 1 items=["HPRI"=1, "LPRI"=0] ("priority")
        # "//读取配置文件"
        n172 = call "Enqueue Element Array.vi"("priority"=w618, "queue index"=1, "error in"=w620, "master data"="" ("Element 1"), "queue in"=w624) -> ("error out"=w623:errorcluster)  [unwired: 5 in, 1 out]
      }
      frame "*Emergency alarm" {
        w633 = u16 1 items=["HPRI"=1, "LPRI"=0] ("priority")
        w634 = u16 1 items=["HPRI"=1, "LPRI"=0] ("priority")
        # "发出处理急停信号的命令"
        # "发出处理急停信号的命令"
        n173 = call "Enqueue Element Array.vi"("priority"=w633, "queue index"=0, "error in"=w627, "master data"="" ("Element 1"), "queue in"=w630) -> ("error out"=w628:errorcluster, "queue out"=w629:T4)  [unwired: 5 in]
        n174 = call "SetTestInfoIndex.vi"("test info index"=13) -> ()
        n175 = call "Enqueue Element Array.vi"("priority"=w634, "queue index"=1, "error in"=w628, "master data"="" ("Element 1"), "queue in"=w629) -> ("error out"=w638:errorcluster)  [unwired: 5 in, 1 out]
      }
    }
    n176 = Wait (ms)(milliseconds to wait=w235) -> ()  [unwired: 1 out]
  }
  n177 = call "Release Queue Array.vi"("error in"=w4, "queue in"=w2) -> ("error out"=w3:errorcluster)  [unwired: 2 in, 3 out]
  n178 = call "Release Queue Array.vi"("error in"=w6, "queue in"=w2) -> ("error out"=w9:errorcluster)  [unwired: 2 in, 3 out]
  n179 = call "MergeErrors.vi"("error in 3 (no error)"=w3, "error in 4 (no error)"=w9) -> ("error out"=w8:errorcluster)  [unwired: 6 in]
  n180 = disable-structure shown="启用" {
    disable-tunnel: w8 -> [w641 w642]
    disable-tunnel: [w640 w642] -> w7
    frame Disabled {
      n181 = call "ExitAppMode.vi"("error in (no error)"=w641) -> ("error out"=w640:errorcluster)  [unwired: 10 in]
    }
    frame Enabled {
    }
  }
  n182 = call <vilib>:"Clear Errors.vi"("error in (no error)"=w7) -> ()  [unwired: 5 in, 2 out]
